vi "S2C_ExeScriptRetest.vi"(8 "Error In":errorcluster, 11 "Q-Ref":refnum<queue>) -> (0 "Error Out":errorcluster)   [LabVIEW 2015]
doc: "Advances the executable script to the next step."
uses:
  Controls/S2C_ResultStatus.ctl
  Globals/S2C_Globals.vi
  LVIS/Sub VIs/Globals/LVIS_IsGlobal.vi
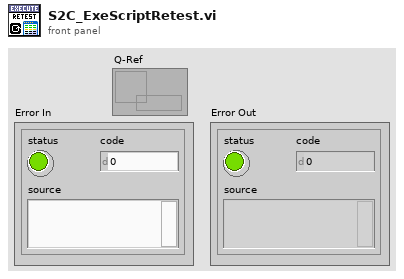
[diagram p1: front panel]
types:
  T1 = typedef "S2C_ResultStatus.ctl" = enum16{"Passed", "Failed", "Logged", "Aborted", "Error", "Testing...", "Paused", "No Record"}
  T2 = cluster{"EventStatus":string, "TestStatus":string, "MeasStatus":string}
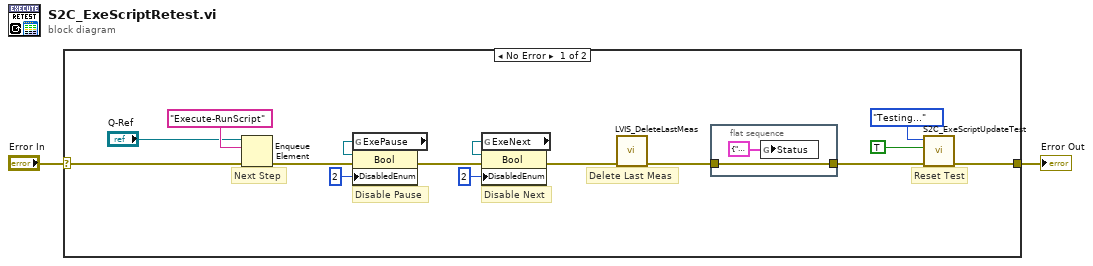
[diagram p0: block diagram]
diagram:
  n1 = case shown="No Error" "Error In" {
    selector: "Error In" -> [w15 w20]
    tunnel: [w7 w20] -> w1
    frame No Error {
      # "Reset Test"
      # "Delete Last Meas"
      # "Disable Pause"
      # "Disable Next"
      # "Next Step"
      n2 = Enqueue Element(queue="Q-Ref", element="Execute-RunScript", error in (no error)=w15) -> (error out=w9:errorcluster)  [unwired: 1 in, 2 out]
      n3 = global read "S2C_Globals.vi" "ExePause"() -> (w11:refnum<vi>)
      n4 = property on="Property Node" class="Bool"(reference=w11, error in=w9, "DisabledEnum"=u8 2) -> (error out=w10:errorcluster)  [unwired: 1 out]
      n5 = global read "S2C_Globals.vi" "ExeNext"() -> (w14:refnum<vi>)
      n6 = property on="Property Node" class="Bool"(reference=w14, error in=w10, "DisabledEnum"=u8 2) -> (error out=w8:errorcluster)  [unwired: 1 out]
      n7 = call "LVIS_DeleteLastMeas.vi"("Error In"=w8) -> ("Error Out"=w5:errorcluster)  [unwired: 10 in]
      n8 = flat-sequence {
        tunnel: w5 -> [w19]
        tunnel: [w19] -> w4
        frame #0 {
          n9 = global write "LVIS_IsGlobal.vi" "Status"(T2 {"EventStatus"="Testing...", "TestStatus"="Testing...", "MeasStatus"="Testing..."} ("Status")) -> ()
        }
      }
      n10 = call "S2C_ExeScriptUpdateTest.vi"("Error In"=w4, "LastMeas?"=TRUE, "Status"=S2C_ResultStatus."Testing...") -> ("Error Out"=w7:errorcluster)  [unwired: 8 in]
    }
    frame Error {
    }
  }
  "Error Out" <- w1
